vi "tcp_concept.vi"() -> ()   [LabVIEW 2014]
panel:
  out "Return Values":u8[](array[numeric])
  in  "Timeout":i32=1000
  in  "Close":bool
  in  "Value":u8
  out "Value":u8
  in  "Write Value":bool
  in  "Read Value":bool
  in  "IP Address":string="127.0.0.1"
  in  "Open Connection":bool
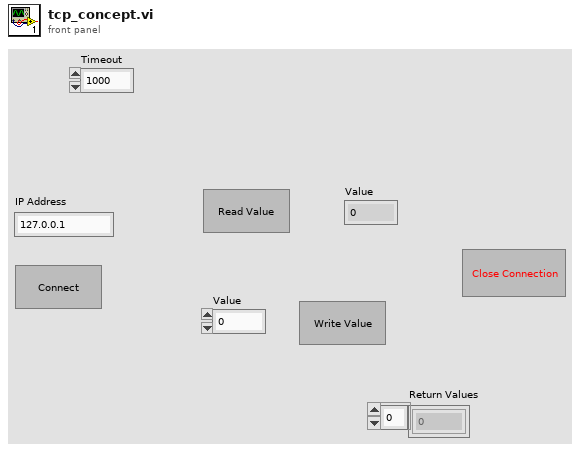
[diagram p1: front panel]
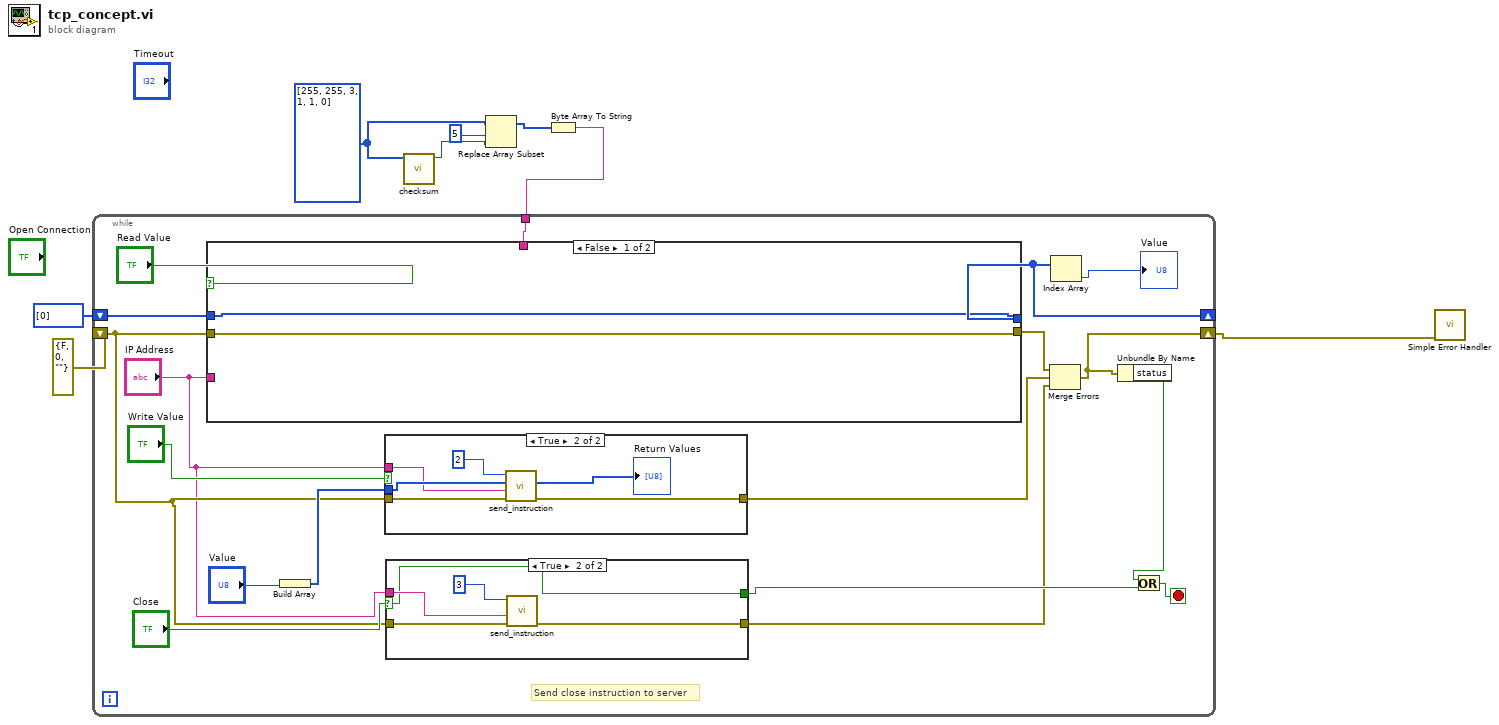
[diagram p0: block diagram]
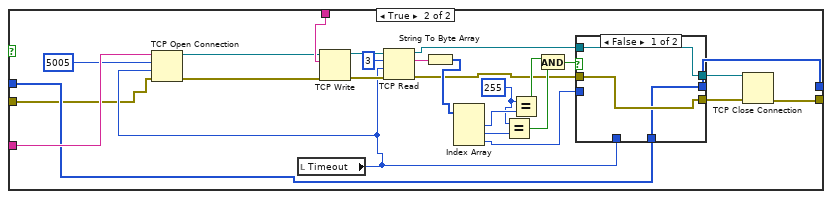
[diagram p4: hidden frame]
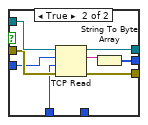
[diagram p5: hidden frame]
diagram:
  w6 = u8[] [255, 255, 3, 1, 1, 0]
  n1 = call "checksum.vi"("Array"=w6) -> ("unsigned 8bit integer"=w7:u8)  [unwired: 10 in]
  n2 = Replace Array Subset(array=w6, new element=w7, index=5) -> (w4:u8[])
  n3 = Byte Array To String(unsigned byte array=w4) -> (string=w3:string)
  n4 = while {
    tunnel: w3 -> [w25]
    shift-right: [w21] -> _
    shift-left: u8[] [0] ("unsigned byte array") -> [w20]
    shift-right: [w14] -> w8
    shift-left: errorcluster {"status"=FALSE, "code"=0, "source"=""} ("error out") -> [w12]
    stop <- w24 stop-if-true
    # "Send close instruction to server"
    n5 = case shown="False" "Read Value" {
      tunnel: w25 -> [_ w68]
      tunnel: [w41 w45] -> w15
      tunnel: [w42 w53] -> w21
      tunnel: "IP Address" -> [_ w50]
      tunnel: w20 -> [w42 w44]
      tunnel: w12 -> [w41 w43]
      frame False {
      }
      frame True {
        w60 = u8 255
        n6 = local read "Timeout"() -> (w49:i32)
        n7 = TCP Open Connection(address=w50, remote port or service name=u16 5005, timeout ms (60000)=w49, error in (no error)=w43) -> (connection ID=w52:refnum<k5>, error out=w51:errorcluster)  [unwired: 1 in]
        n8 = TCP Write(connection ID=w52, data in=w68, error in (no error)=w51) -> (connection ID out=w67:refnum<k5>, error out=w66:errorcluster)  [unwired: 1 in, 1 out]
        n9 = TCP Read(connection ID=w67, bytes to read=3, error in (no error)=w66, 9:w49) -> (connection ID out=w55:refnum<k5>, data out=w64:string, error out=w56:errorcluster)  [unwired: 1 in]
        n10 = String To Byte Array(string=w64) -> (unsigned byte array=w63:u8[])
        n11 = Index Array(array=w63) -> (element #1=w62:u8, element #2=w61:u8, element #3=w54:u8)  [unwired: 3 in]
        n12 = Equal?(x=w60, y=w61) -> (x = y?=w57:bool)
        n13 = Equal?(x=w60, y=w62) -> (x = y?=w58:bool)
        n14 = And(x=w58, y=w57) -> (x .and. y?=w59:bool)
        n15 = case shown="False" w59 {
          tunnel: w56 -> [w71 w78]
          tunnel: w55 -> [w70 w79]
          tunnel: w54 -> [_ w77]
          tunnel: w49 -> [_ w76]
          tunnel: [w71 w75] -> w46
          tunnel: [w70 w74] -> w47
          tunnel: [w69 w72] -> w53
          tunnel: w44 -> [w69 _]
          frame False {
          }
          frame True {
            n16 = TCP Read(connection ID=w79, bytes to read=w77, error in (no error)=w78, 9:w76) -> (connection ID out=w74:refnum<k5>, data out=w73:string, error out=w75:errorcluster)  [unwired: 1 in]
            n17 = String To Byte Array(string=w73) -> (unsigned byte array=w72:u8[])
          }
        }
        n18 = TCP Close Connection(connection ID=w47, error in (no error)=w46) -> (error out=w45:errorcluster)  [unwired: 1 in, 1 out]
      }
    }
    n19 = Build Array("Value") -> (w17:u8[])
    n20 = case shown="True" "Write Value" {
      tunnel: w17 -> [_ w39]
      tunnel: "IP Address" -> [_ w38]
      tunnel: w12 -> [w34 w37]
      tunnel: [w34 w36] -> w16
      frame False {
      }
      frame True {
        n21 = call "send_instruction.vi"("error in"=w37, "IP Address"=w38, "Parameters"=w39, "Instruction"=u8 2) -> ("error out"=w36:errorcluster, "Return Values"=→"Return Values":u8[])  [unwired: 6 in]
      }
    }
    n22 = case shown="True" "Close" {
      selector: "Close" -> [w27 w29]
      tunnel: "IP Address" -> [_ w32]
      tunnel: w12 -> [w28 w31]
      tunnel: [w28 w30] -> w9
      tunnel: [w27 w29] -> w10
      frame False {
      }
      frame True {
        n23 = call "send_instruction.vi"("error in"=w31, "IP Address"=w32, "Instruction"=u8 3) -> ("error out"=w30:errorcluster)  [unwired: 7 in, 1 out]
      }
    }
    n24 = Merge Errors(w15, w16, w9) -> (w14:errorcluster)
    n25 = Index Array(array=w21) -> (element=→"Value":u8)  [unwired: 1 in]
    n26 = Unbundle By Name(w14) -> ("status"=w23:bool)
    n27 = Or(x=w23, y=w10) -> (x .or. y?=w24:bool)
  }
  n28 = call <vilib>:"Simple Error Handler.vi"("error in (no error)"=w8) -> ()  [unwired: 4 in, 5 out]
